vi "Calculate_Proper_Divisors.vi"(11 "Input Integer":i32) -> (1 "List of Divisors":i32[](array[numeric]), 3 "Sum of Divisors":i32)   [LabVIEW 2026]
panel:
  # "METHOD - 3 : WITH SHIFT REGISTERS"
  # "proper divisors of an integer"
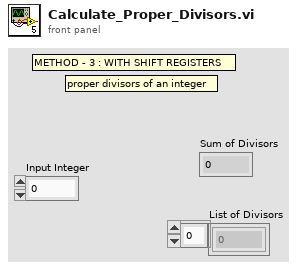
[diagram p1: front panel]
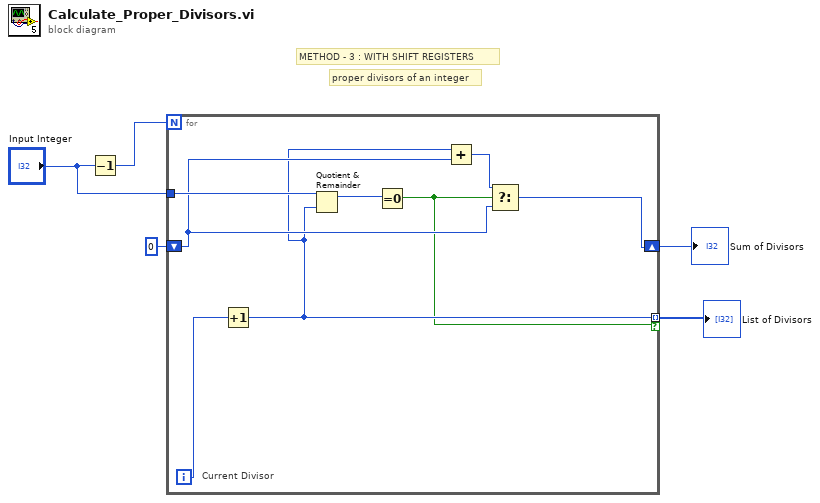
[diagram p0: block diagram]
diagram:
  # "METHOD - 3 : WITH SHIFT REGISTERS"
  # "proper divisors of an integer"
  n1 = Decrement(x="Input Integer") -> (x-1=w5:i32)
  n2 = for {
    N: w5 -> [_]
    tunnel: "Input Integer" -> [w11]
    shift-right: [w8] -> w2
    shift-left: 0 -> [w9]
    tunnel: [w7] -> w1 mode=indexing if=w6
    i -> [w12]
    # "Current Divisor"
    n3 = Increment(x=w12) -> (x+1=w7:i32)
    n4 = Quotient & Remainder(x=w11, y=w7) -> (x-y*floor(x/y)=w13:i32)  [unwired: 1 out]
    n5 = Equal To 0?(x=w13) -> (x = 0?=w6:bool)
    n6 = Add(x=w7, y=w9) -> (x+y=w10:i32)
    n7 = Select(t=w10, s=w6, f=w9) -> (s? t:f=w8:i32)
  }
  "Sum of Divisors" <- w2
  "List of Divisors" <- w1
